vi "table.vi"() -> ()   [LabVIEW 2015]
panel:
  in  "no.":dbl
  out "Result":dbl
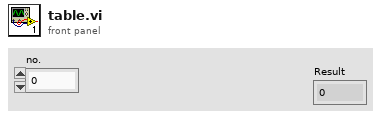
[diagram p1: front panel]
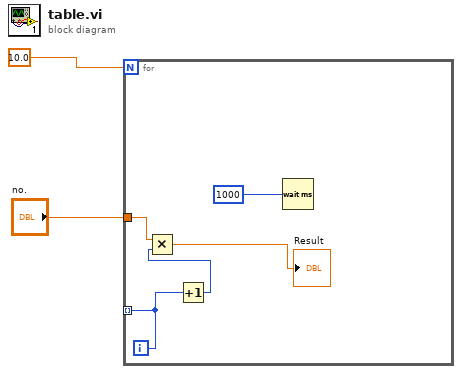
[diagram p0: block diagram]
diagram:
  n1 = for {
    N: 10.0 ("Numeric") -> [_]
    tunnel: "no." -> [w5]
    tunnel: [w3] -> _ mode=indexing
    i -> [w3]
    n2 = Increment(x=w3) -> (x+1=w4:i32)
    n3 = Multiply(x=w5, y=w4) -> (x*y=→"Result":dbl)
    n4 = Wait (ms)(milliseconds to wait=u32 1000) -> ()  [unwired: 1 out]
  }
